vi "Filter.vi"(9 "data":dbl, 10 "Buffer Len":i32=10, 11 "Buffer in":dbl[](array[numeric])) -> (2 "ave out":dbl, 3 "Buffer out":dbl[](array[numeric]))   [LabVIEW 2019]
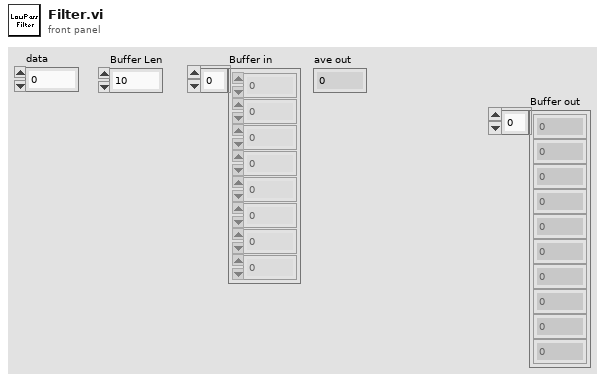
[diagram p1: front panel]
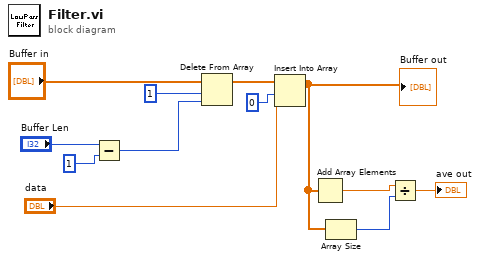
[diagram p0: block diagram]
diagram:
  n1 = Subtract(x="Buffer Len", y=1) -> (x-y=w3:i32)
  n2 = Delete From Array(array="Buffer in", length=1, index=w3) -> (array with subset deleted=w2:dbl[])  [unwired: 1 out]
  n3 = Insert Into Array(array=w2, index=0, new element="data") -> (w7:dbl[])
  "Buffer out" <- w7
  n4 = Add Array Elements(numeric array=w7) -> (sum=w10:dbl)
  n5 = Array Size(array=w7) -> (size(s)=w9:i32)
  n6 = Divide(x=w10, y=w9) -> (x/y=→"ave out":dbl)
